vi "AM_Talk_To_Board.vi"() -> ()   [LabVIEW 2019]
doc: "Emulate a Serial Console. \n\nSend Commands that alter board state using Write CMD (No data is read from board)\n\nSend Commands to Read Data from board using Write / Read\n\nR. Sheehan 28 - 1 - 2021"
uses:
  <vilib>/Instr/_visa.llb/VISA Configure Serial Port (Instr).vi
panel:
  in  "Tab Control":enum32{"Comms", "Commands", "Clusters"}(tab)
  in  "Addr":refnum<visa-resource-name>
  in  "Open Comms":bool
  out "Addr 2":refnum<visa-resource-name>
  out "Open":bool
  in  "Write CMD":bool
  in  "Write / Read":bool
  in  "Write Only":string
  in  "Write and Read":string
  out "Output":string
  out "Bytes":u32
  out "error out":errorcluster
  in  "Stop":bool
  # "Sketch DCWriteRead.ino\n\nCommands \n\nOutput Voltage on ChA: a<val>\n\nOutput Voltage on ChB: b<val>\n\nRead Voltages on A0 - A5: l"
  # "Sketch: SigGenWriteRead.ino\n\nCommands \n\nChange Frequency: w<val>\n\nRead Vpp on A0 and A1: r"
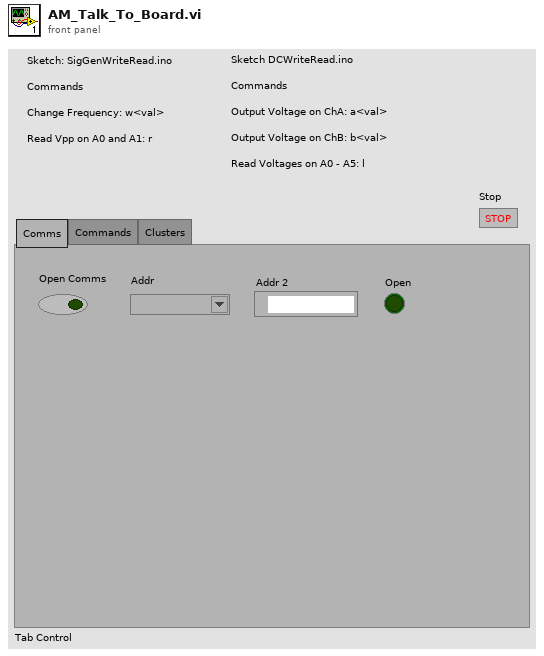
[diagram p1: front panel]
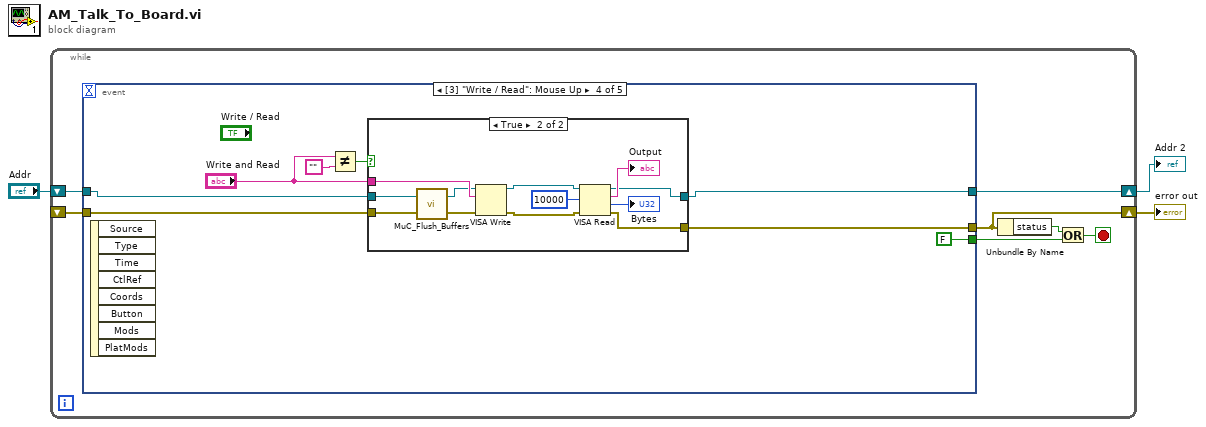
[diagram p0: block diagram]
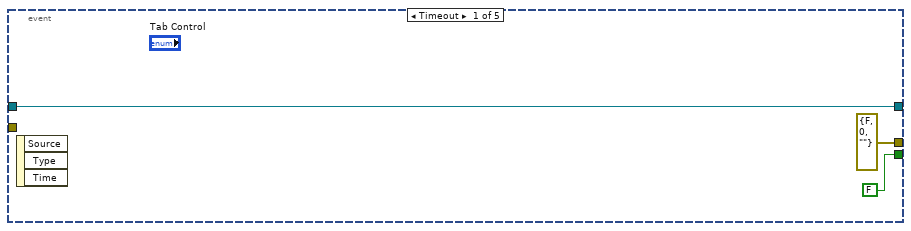
[diagram p2: hidden frame]
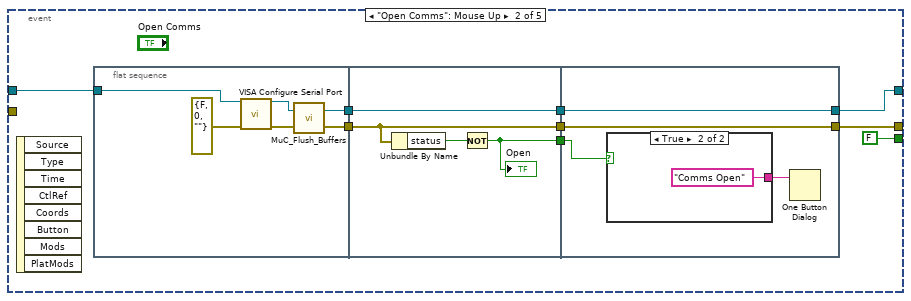
[diagram p3: hidden frame]
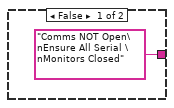
[diagram p4: hidden frame]
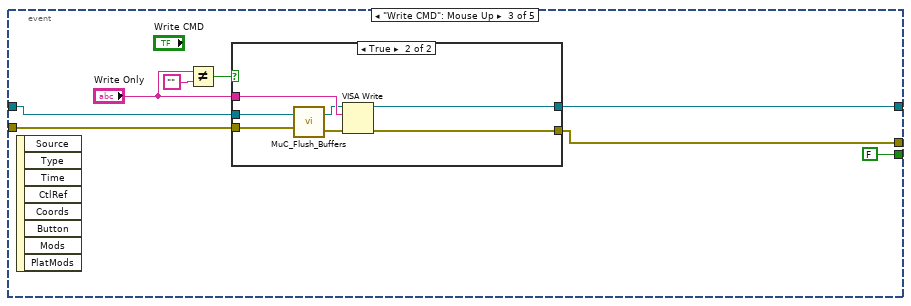
[diagram p5: hidden frame]
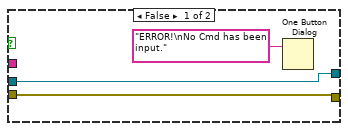
[diagram p6: hidden frame]
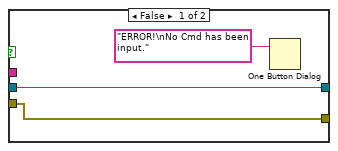
[diagram p7: hidden frame]
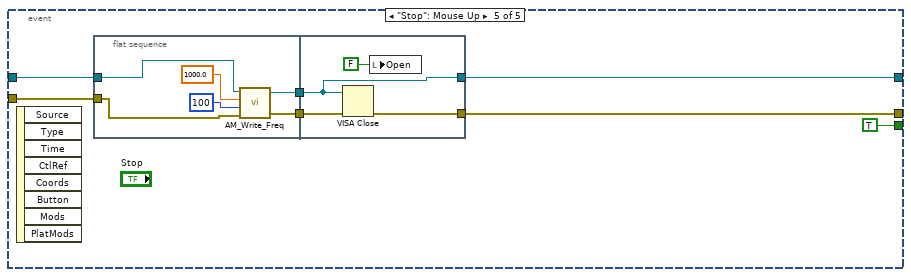
[diagram p8: hidden frame]
diagram:
  n1 = while {
    shift-right: [w9] -> w2
    shift-left: "Addr" -> [w10]
    shift-right: [w8] -> w1
    shift-left: _ -> [w7]
    stop <- w5 stop-if-true
    n2 = event shown="[3] \"Write / Read\": Mouse Up" {
      selector: _ -> [_ _ _ _ _]
      dyn-events: _ -> [_ _ _ _ _]
      timeout: _ -> [_ _ _ _ _]
      tunnel: w10 -> [w11 w22 w40 w61 w83]
      tunnel: [w11 w20 w41 w59 w81] -> w9
      tunnel: [errorcluster {"status"=FALSE, "code"=0, "source"=""} ("error in (no error)") w17 w42 w58 w85] -> w8
      tunnel: w7 -> [_ _ w43 w60 w84]
      tunnel: [FALSE FALSE FALSE FALSE TRUE] -> w4
      event Timeout {
        n3 = event-data() -> ()  [unwired: 1 in, 3 out]
      }
      event "Open Comms": Mouse Up {
        n4 = event-data() -> ()  [unwired: 1 in, 8 out]
        n5 = flat-sequence {
          tunnel: w22 -> [w27]
          tunnel: [w25] -> w19
          tunnel: [w23] -> w18
          tunnel: w19 -> [w32]
          tunnel: w18 -> [w31]
          tunnel: [w32] -> w16
          tunnel: [w31] -> w15
          tunnel: [w29] -> w14
          tunnel: [w35] -> w17
          tunnel: [w36] -> w20
          tunnel: w16 -> [w36]
          tunnel: w15 -> [w35]
          tunnel: w14 -> [w34]
          frame #0 {
            n6 = call-poly "VISA Configure Serial Port"("VISA resource name"=w27, "error in (no error)"=errorcluster {"status"=FALSE, "code"=0, "source"=""}) -> ("VISA resource name out"=w26:refnum<visa-resource-name>, "error out"=w24:errorcluster)  [unwired: 7 in, 5 out]
            n7 = call "MuC_Flush_Buffers.vi"("error in (no error)"=w24, "VISA resource name"=w26) -> ("error out"=w23:errorcluster, "VISA resource name 2"=w25:refnum<visa-resource-name>)
          }
          frame #1 {
            n8 = Unbundle By Name(w31) -> ("status"=w30:bool)
            n9 = Not(x=w30) -> (.not. x?=w29:bool)
            "Open" <- w29
          }
          frame #2 {
            n10 = case shown="True" w34 {
              tunnel: ["Comms NOT Open\nEnsure All Serial \nMonitors Closed" ("message") "Comms Open" ("message")] -> w33
              frame False {
              }
              frame True {
              }
            }
            n11 = One Button Dialog(message=w33) -> ()  [unwired: 1 in, 1 out]
          }
        }
      }
      event "Write CMD": Mouse Up {
        n12 = event-data() -> ()  [unwired: 1 in, 8 out]
        n13 = Not Equal?(x="Write Only", y="") -> (x != y?=w45:bool)
        n14 = case shown="True" w45 {
          tunnel: "Write Only" -> [_ w56]
          tunnel: w43 -> [w47 w51]
          tunnel: [w47 w55] -> w42
          tunnel: [w48 w54] -> w41
          tunnel: w40 -> [w48 w53]
          frame False {
            n15 = One Button Dialog(message="ERROR!\nNo Cmd has been input.") -> ()  [unwired: 1 in, 1 out]
          }
          frame True {
            n16 = call "MuC_Flush_Buffers.vi"("error in (no error)"=w51, "VISA resource name"=w53) -> ("error out"=w50:errorcluster, "VISA resource name 2"=w52:refnum<visa-resource-name>)
            n17 = VISA Write(VISA resource name=w52, write buffer=w56, error in (no error)=w50) -> (VISA resource name out=w54:refnum<visa-resource-name>, error out=w55:errorcluster)  [unwired: 1 out]
          }
        }
      }
      event "Write / Read": Mouse Up {
        n18 = event-data() -> ()  [unwired: 1 in, 8 out]
        n19 = Not Equal?(x="Write and Read", y="") -> (x != y?=w63:bool)
        n20 = case shown="True" w63 {
          tunnel: "Write and Read" -> [_ w75]
          tunnel: w61 -> [w66 w71]
          tunnel: w60 -> [w65 w69]
          tunnel: [w66 w73] -> w59
          tunnel: [w65 w72] -> w58
          frame False {
            n21 = One Button Dialog(message="ERROR!\nNo Cmd has been input.") -> ()  [unwired: 1 in, 1 out]
          }
          frame True {
            n22 = call "MuC_Flush_Buffers.vi"("error in (no error)"=w69, "VISA resource name"=w71) -> ("error out"=w68:errorcluster, "VISA resource name 2"=w70:refnum<visa-resource-name>)
            n23 = VISA Write(VISA resource name=w70, write buffer=w75, error in (no error)=w68) -> (VISA resource name out=w78:refnum<visa-resource-name>, error out=w79:errorcluster)  [unwired: 1 out]
            n24 = VISA Read(VISA resource name=w78, byte count=u32 10000, error in (no error)=w79) -> (VISA resource name out=w73:refnum<visa-resource-name>, read buffer=→"Output":string, return count=→"Bytes":u32, error out=w72:errorcluster)
          }
        }
      }
      event "Stop": Mouse Up {
        n25 = event-data() -> ()  [unwired: 1 in, 8 out]
        n26 = flat-sequence {
          tunnel: w84 -> [w89]
          tunnel: w83 -> [w92]
          tunnel: [w91] -> w82
          tunnel: [w90] -> w80
          tunnel: [w96] -> w85
          tunnel: w82 -> [w94]
          tunnel: [w94] -> w81
          tunnel: w80 -> [w93]
          frame #0 {
            n27 = call "AM_Write_Freq.vi"("error in (no error)"=w89, "Delay / ms"=u32 100, "f / Hz"=1000.0, "VISA resource name"=w92) -> ("error out"=w90:errorcluster, "VISA resource name 2"=w91:refnum<visa-resource-name>)  [unwired: 1 out]
          }
          frame #1 {
            n28 = VISA Close(VISA resource name=w94, error in (no error)=w93) -> (error out=w96:errorcluster)
            n29 = local write "Open"(FALSE) -> ()
          }
        }
      }
    }
    n30 = Unbundle By Name(w8) -> ("status"=w6:bool)
    n31 = Or(x=w6, y=w4) -> (x .or. y?=w5:bool)
  }
  "Addr 2" <- w2
  "error out" <- w1
